vi "Tokenize.vi"(11 "string":string) -> (3 "tokens":string[](array[string]))   [LabVIEW 2017]
doc: "Separates <b>string</b> into array of <b>tokens</b>."
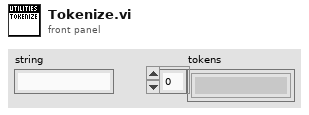
[diagram p1: front panel]
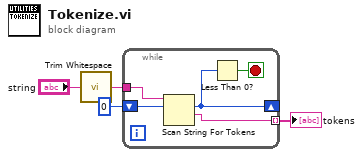
[diagram p0: block diagram]
diagram:
  n1 = call <vilib>:"Trim Whitespace.vi"("string"="string") -> ("trimmed string"=w1:string)  [unwired: 1 in]
  n2 = while {
    tunnel: w1 -> [w9]
    tunnel: [w7] -> w3 mode=indexing
    shift-right: [w6] -> _
    shift-left: 0 ("offset past token") -> [w8]
    stop <- w5 stop-if-true
    n3 = Scan String For Tokens(8:w8, 9:w9) -> (1:w7:string, 2:w6:i32)  [unwired: 4 in, 2 out]
    n4 = Less Than 0?(x=w6) -> (x < 0?=w5:bool)
  }
  "tokens" <- w3
